vi "WebDav FGV.vi"(0 "State":T4, 5 "RT (Source) Location":string, 7 "Parent":string, 9 "Local (Destination) Folder":path, 11 "error in (no error)":errorcluster) -> (3 "Download Progress":u64(slide) max=195 scale=0.0..100.0, 4 "Directory Listing":T2, 8 "Event":T3(ring), 10 "Local (Destination) Folder Out":path, 15 "error out":errorcluster)   [LabVIEW 2017]
uses:
  controls/WebDav Enum Ring.ctl
  <vilib>/WebDAVClient/Advanced/FileInfo.ctl
  <vilib>/WebDAVClient/Advanced/Multi Event/Asynchronous Get File.vi
  <vilib>/WebDAVClient/NI_WebDAV.lvlib
panel:
  in  "file info":T1
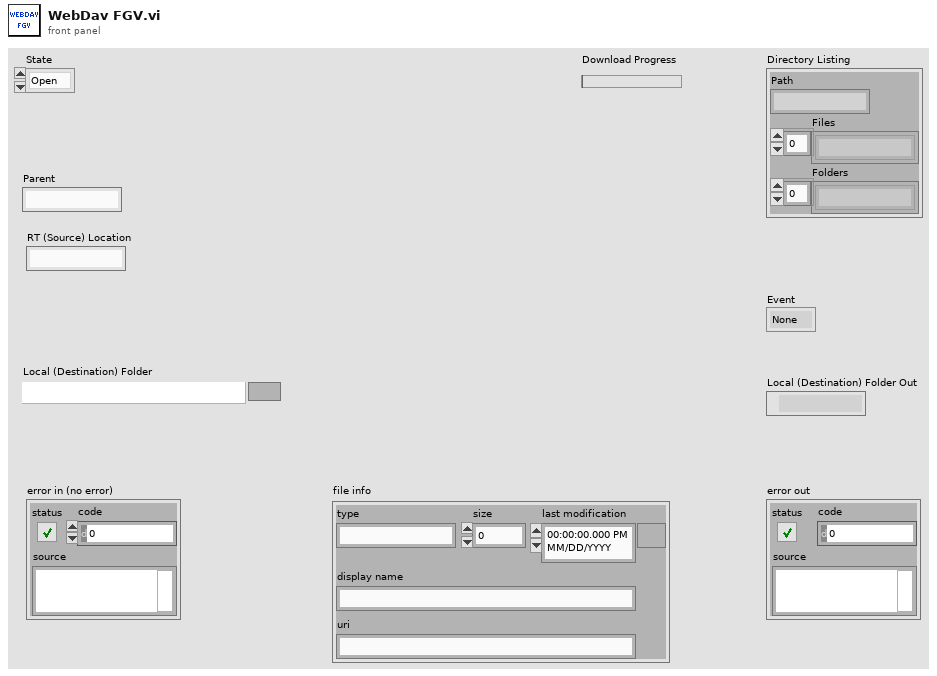
[diagram p1: front panel]
types:
  T1 = typedef "NI_WebDAV.lvlib/FileInfo.ctl" = cluster{"type":string, "size":u64, "last modification":timestamp, "display name":string, "uri":string}
  T2 = cluster{"Path":string, "Files":string[], "Folders":string[]}
  T3 = enum16{"None", "List Complete", "File Transfer Complete"}
  T4 = typedef "WebDav Enum Ring.ctl" = enum16{"Open", "Close", "List Directory", "Get File", "Cancel File Request", "Handle Events"}
  T5 = typedef "NI_WebDAV.lvlib/Asynchronous Session Handle.ctl" = refnum<k1>
  T6 = typedef "NI_WebDAV.lvlib/Asynchronous Request Handle.ctl" = refnum<k1>
  T7 = typedef "NI_WebDAV.lvlib/Request Status.ctl" = enum16{"working", "complete", "aborted", "timeout", "error"}
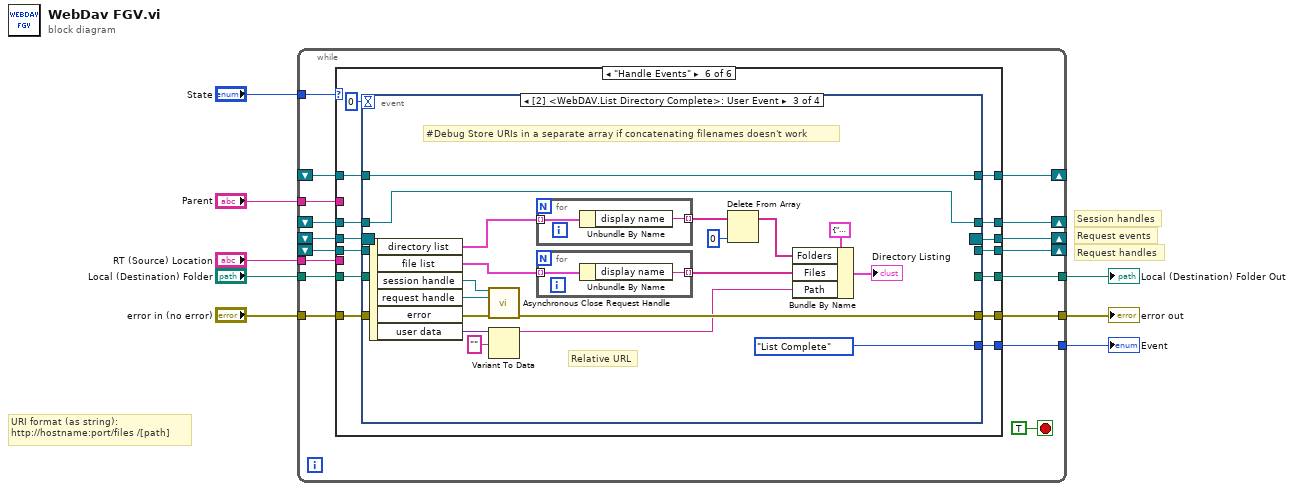
[diagram p0: block diagram]
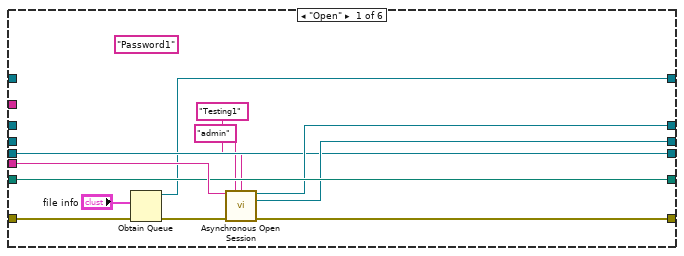
[diagram p2: hidden frame]
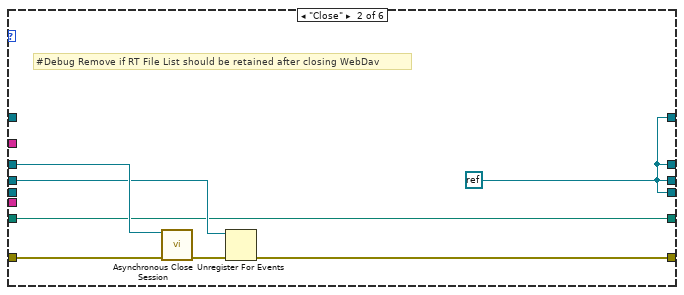
[diagram p3: hidden frame]
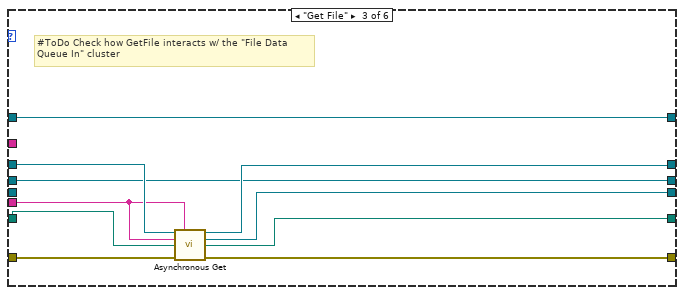
[diagram p4: hidden frame]
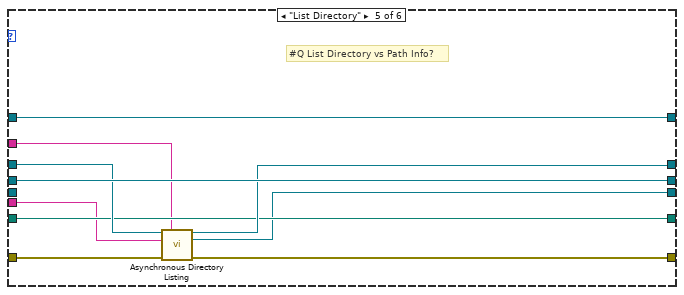
[diagram p6: hidden frame]
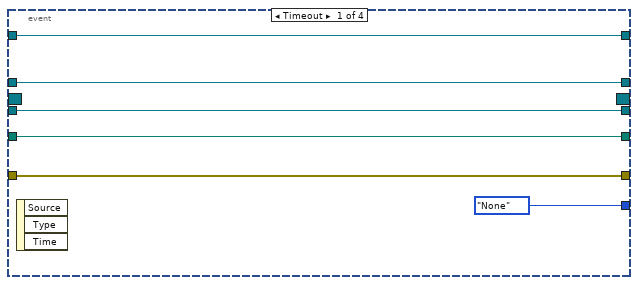
[diagram p7: hidden frame]
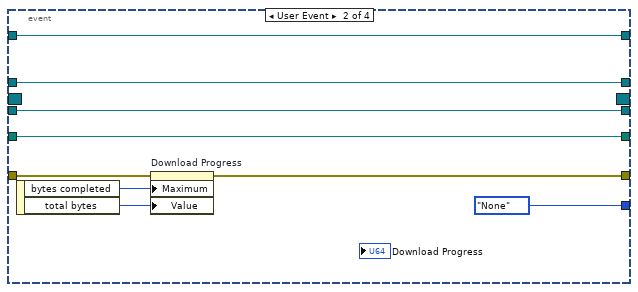
[diagram p8: hidden frame]
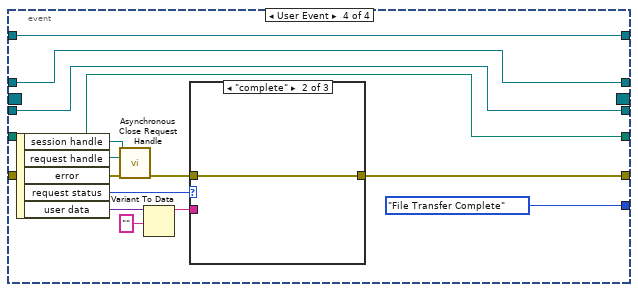
[diagram p9: hidden frame]
diagram:
  # "Request handles"
  # "URI format (as string):\nhttp://hostname:port/files /[path]"
  # "Request events"
  # "Session handles"
  n1 = while {
    tunnel: "error in (no error)" -> [w25]
    tunnel: [w11] -> w5
    tunnel: "State" -> [w24]
    tunnel: "RT (Source) Location" -> [w23]
    shift-right: [w22] -> _
    shift-left: _ -> [w21]
    tunnel: "Local (Destination) Folder" -> [w20]
    shift-right: [w19] -> _
    shift-left: _ -> [w18]
    tunnel: [w17] -> w3
    shift-right: [w15] -> _
    shift-left: _ -> [w16]
    tunnel: [w14] -> w2
    shift-right: [w13] -> _
    shift-left: _ -> [w12]
    tunnel: "Parent" -> [w9]
    stop <- TRUE stop-if-true
    n2 = case shown="\"Handle Events\"" w24 {
      tunnel: w25 -> [w30 w44 w53 w60 w69 w84]
      tunnel: [w37 w41 w54 w60 w68 w83] -> w11
      tunnel: w23 -> [w36 _ w46 _ w63 _]
      tunnel: [w34 w38 w51 w56 w67 w79] -> w22
      tunnel: w21 -> [_ w43 w50 w56 w66 w80]
      tunnel: w20 -> [w35 w39 w52 w58 w64 w82]
      tunnel: [w33 w38 w48 w59 w70 w75] -> w19
      tunnel: w18 -> [_ w40 w48 w59 w70 w76]
      tunnel: [w35 w39 w49 w58 w64 w81] -> w17
      tunnel: w16 -> [_ _ w47 w57 w65 w78]
      tunnel: [w28 w38 w47 w57 w65 w77] -> w15
      tunnel: [_ _ _ _ _ w74] -> w14
      tunnel: [w32 w38 w45 w55 w62 w72] -> w13
      tunnel: w12 -> [w32 _ _ w55 _ w73]
      tunnel: w9 -> [_ _ _ _ w61 _]
      frame "Open" {
        (unwired) "Password1" ("password")
        n3 = Obtain Queue(element data type="file info", error in (no error)=w30) -> (queue out=w28:refnum<queue>, error out=w29:errorcluster)  [unwired: 3 in, 1 out]
        n4 = call <vilib>:"Asynchronous Open Session.vi"("host uri prefix"=w36, "username"="admin", "password"="Testing1", "error in (no error)"=w29) -> ("session handle out"=w34:T5, "Request Events"=w33:refnum<event-registration>, "error out"=w37:errorcluster)  [unwired: 9 in]
      }
      frame "Close" {
        w38 = refnum<k0> refnum
        # "#Debug Remove if RT File List should be retained after closing WebDav"
        n5 = call <vilib>:"Asynchronous Close Session.vi"("session handle"=w43, "error in (no error)"=w44) -> ("error out"=w42:errorcluster)  [unwired: 13 in]
        n6 = Unregister For Events(event registration refnum=w40, error in=w42) -> (error out=w41:errorcluster)
      }
      frame "Get File" {
        # "#ToDo Check how GetFile interacts w/ the \"File Data\nQueue In\" cluster"
        n7 = call-poly <vilib>:"Asynchronous Get.vi"("session handle"=w50, "user data"=w46, "relative uri"=w46, "local file path"=w52, "error in (no error)"=w53) -> ("session handle out"=w51:T5, "request handle out"=w45:T6, "local file path out"=w49:path, "error out"=w54:errorcluster)  [unwired: 7 in]
      }
      frame "Cancel File Request" {
      }
      frame "List Directory" {
        # "#Q List Directory vs Path Info?"
        n8 = call <vilib>:"Asynchronous Directory Listing.vi"("session handle"=w66, "user data"=w61, "relative uri"=w63, "error in (no error)"=w69) -> ("session handle out"=w67:T5, "request handle out"=w62:T6, "error out"=w68:errorcluster)  [unwired: 9 in]
      }
      frame "Handle Events" {
        n9 = event shown="[2] <WebDAV.List Directory Complete>: User Event" {
          selector: w76 -> [_ _ _ _]
          dyn-events: [_ _ _ _] -> w75
          timeout: 0 -> [_ _ _ _]
          tunnel: w84 -> [w90 w97 _ _]
          tunnel: [w90 w96 w113 w131] -> w83
          tunnel: w82 -> [w89 w92 _ w123]
          tunnel: [w89 w92 _ w123] -> w81
          tunnel: w80 -> [w88 w94 w104 w126]
          tunnel: [w88 w94 w104 w126] -> w79
          tunnel: [w87 w95 w112 w127] -> w77
          tunnel: w78 -> [w87 w95 w112 w127]
          tunnel: [T3."None" ("Event") T3."None" ("Event") T3."List Complete" ("Event") T3."File Transfer Complete" ("Event")] -> w74
          tunnel: w73 -> [w86 w93 _ w124]
          tunnel: [w86 w93 _ w124] -> w72
          event Timeout {
            n10 = event-data() -> ()  [unwired: 1 in, 3 out]
          }
          event User Event {
            n11 = event-data() -> ("bytes completed"=w98:u64, "total bytes"=w99:u64)  [unwired: 1 in]
            n12 = property on="Download Progress" class="Slide (strict)"(error in=w97, "Maximum"=w98, "Value"=w99) -> (error out=w96:errorcluster)  [unwired: 1 in, 1 out]
          }
          event User Event {
            # "#Debug Store URIs in a separate array if concatenating filenames doesn't work"
            # "Relative URL"
            n13 = event-data() -> ("directory list"=w103:T1[], "file list"=w114:T1[], "session handle"=w116:T5, "request handle"=w117:T6, "error"=w115:errorcluster, "user data"=w111:variant)  [unwired: 1 in]
            n14 = call <vilib>:"Asynchronous Close Request Handle.vi"("session handle"=w116, "request handle"=w117, "error in (no error)"=w115) -> ("error out"=w113:errorcluster)  [unwired: 11 in, 1 out]
            n15 = Variant To Data(type="", Variant=w111) -> (data=w106:string)  [unwired: 1 in, 1 out]
            n16 = for {
              tunnel: w103 -> [w119] mode=indexing
              tunnel: [w118] -> w100 mode=indexing
              n17 = Unbundle By Name(w119) -> ("display name"=w118:string)
            }
            n18 = for {
              tunnel: w114 -> [w121] mode=indexing
              tunnel: [w120] -> w107 mode=indexing
              n19 = Unbundle By Name(w121) -> ("display name"=w120:string)
            }
            n20 = Delete From Array(array=w100, index=0) -> (array with subset deleted=w101:string[])  [unwired: 1 in, 1 out]
            n21 = Bundle By Name(cluster=T2 {"Path"="", "Files"=[], "Folders"=[]}, "Folders"=w101, "Files"=w107, "Path"=w106) -> (→"Directory Listing":T2)
          }
          event User Event {
            n22 = event-data() -> ("session handle"=w128:T5, "request handle"=w135:T6, "error"=w134:errorcluster, "request status"=w133:T7, "user data"=w130:variant)  [unwired: 1 in]
            n23 = call <vilib>:"Asynchronous Close Request Handle.vi"("session handle"=w128, "request handle"=w135, "error in (no error)"=w134) -> ("error out"=w132:errorcluster)  [unwired: 11 in, 1 out]
            n24 = Variant To Data(type="", Variant=w130) -> (data=w129:string)  [unwired: 1 in, 1 out]
            n25 = case shown="\"complete\"" w133 {
              tunnel: w132 -> [w136 w137 w138]
              tunnel: [w136 w137 w138] -> w131
              tunnel: w129 -> [_ _ _]
              frame "working", Default {
              }
              frame "complete" {
              }
              frame "aborted" {
                # "#ToDo Remove temp file"
              }
            }
          }
        }
      }
    }
  }
  "error out" <- w5
  "Local (Destination) Folder Out" <- w3
  "Event" <- w2
